vi "数字量输入自动检测.vi"(10 "选择?":bool) -> ()   [LabVIEW 2010]
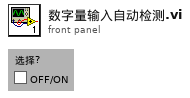
[diagram p1: front panel]
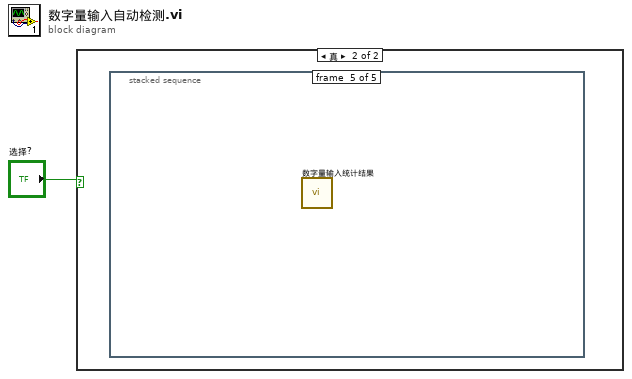
[diagram p0: block diagram]
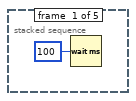
[diagram p3: hidden frame]
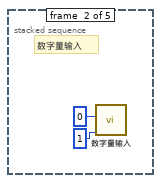
[diagram p4: hidden frame]
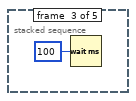
[diagram p5: hidden frame]
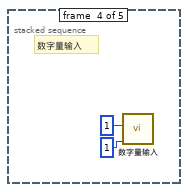
[diagram p6: hidden frame]
diagram:
  n1 = case shown="真" "选择?" {
    frame False {
    }
    frame True {
      n2 = stacked-sequence {
        frame #0 {
          n3 = Wait (ms)(milliseconds to wait=u32 100 ("等待时间（毫秒）")) -> ()  [unwired: 1 out]
        }
        frame #1 {
          # "数字量输入"
          n4 = call "数字量输入.vi"("CAN端口"=u16 1, "输入值"=i16 0) -> ()  [unwired: 10 in]
        }
        frame #2 {
          n5 = Wait (ms)(milliseconds to wait=u32 100 ("等待时间（毫秒）")) -> ()  [unwired: 1 out]
        }
        frame #3 {
          # "数字量输入"
          n6 = call "数字量输入.vi"("CAN端口"=u16 1, "输入值"=i16 1) -> ()  [unwired: 10 in]
        }
        frame #4 {
          n7 = call "数字量输入统计结果.vi"() -> ()  [unwired: 12 in]
        }
      }
    }
  }
